vi "Read Temperature Data.vi"(4 "PROM correction Values":u16[](array[numeric]), 6 "I2C Slave Address":u8=119 format="%x", 7 "I2C Channel":u8, 8 "Error In":errorcluster, 11 "LINX Resource in":T1) -> (0 "Error Out":errorcluster, 2 "dT":i32, 3 "LINX Resource out":T1, 5 "Temp":dbl format="%.2g")   [LabVIEW 2014]
uses:
  <vilib>/MakerHub/LINX/Private/Type Defs/LINX Ref.ctl
  <vilib>/MakerHub/LINX/Private/Type Defs/Platform.ctl
  <vilib>/MakerHub/LINX/Private/Type Defs/Interface.ctl
  <vilib>/MakerHub/LINX/Private/Device/Type Defs/LINX Device Config.ctl
  <vilib>/MakerHub/LINX/Private/Device/Type Defs/TCP Config.ctl
  <vilib>/MakerHub/LINX/Private/Device/Type Defs/Channels.ctl
  <vilib>/MakerHub/LINX/Private/Local IO/LinxI2cWrite.vi
  <vilib>/MakerHub/LINX/Public/Utilities/Check Channel.vi
  <vilib>/MakerHub/LINX/Private/Utilties/Generate Error.vi
  <vilib>/MakerHub/LINX/LMH-LINX.lvlib
  <vilib>/MakerHub/LINX/Private/Device/Device.lvlib
panel:
  out "C6":u16
  out "C5":u16
  out "D2":u32
  out "D2 Raw Data Values":u16[](array[numeric])
  # "Data 23-16"
  # "Data 8-15"
  # "Datas 0-7"
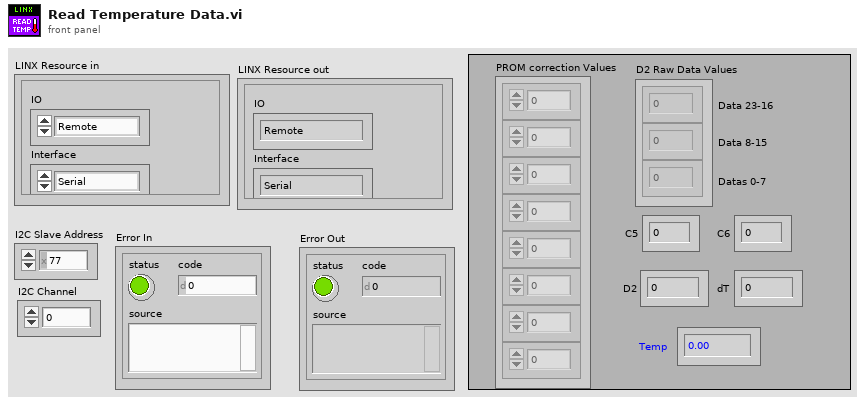
[diagram p1: front panel]
types:
  T1 = typedef "LMH-LINX.lvlib/LINX Ref.ctl" = cluster{"IO":T2, "Interface":T3, "LINX Device Config":T4}
  T2 = typedef "LMH-LINX.lvlib/Platform.ctl" = enum16{"Remote", "Local"}
  T3 = typedef "LMH-LINX.lvlib/Interface.ctl" = enum16{"Serial", "TCP"}
  T4 = typedef "LMH-LINX.lvlib/Device.lvlib/LINX Device Config.ctl" = cluster{"Interface":T3, "COM Port":refnum<visa-resource-name>, "TCP Configuration":T5, "Device Family":u8, "Device ID":u8, "Device Name":string, "TCP Ref":refnum<k5>, "Channels":T6}
  T5 = typedef "LMH-LINX.lvlib/Device.lvlib/TCP Config.ctl" = cluster{"IP Address":string, "Port":u16}
  T6 = typedef "LMH-LINX.lvlib/Channels.ctl" = cluster{"DI":u8[], "DO":u8[], "AI":u8[], "AO":u8[], "PWM":u8[], "QE":u8[], "UART":u8[], "I2C 2":u8[], "SPI":u8[], "CAN":u8[], "Servo":u8[], "AI Ref (V)":dbl, "AI Resolution (Bits)":u8, "AO Ref (V)":dbl, "AO Resolution (Bits)":u8}
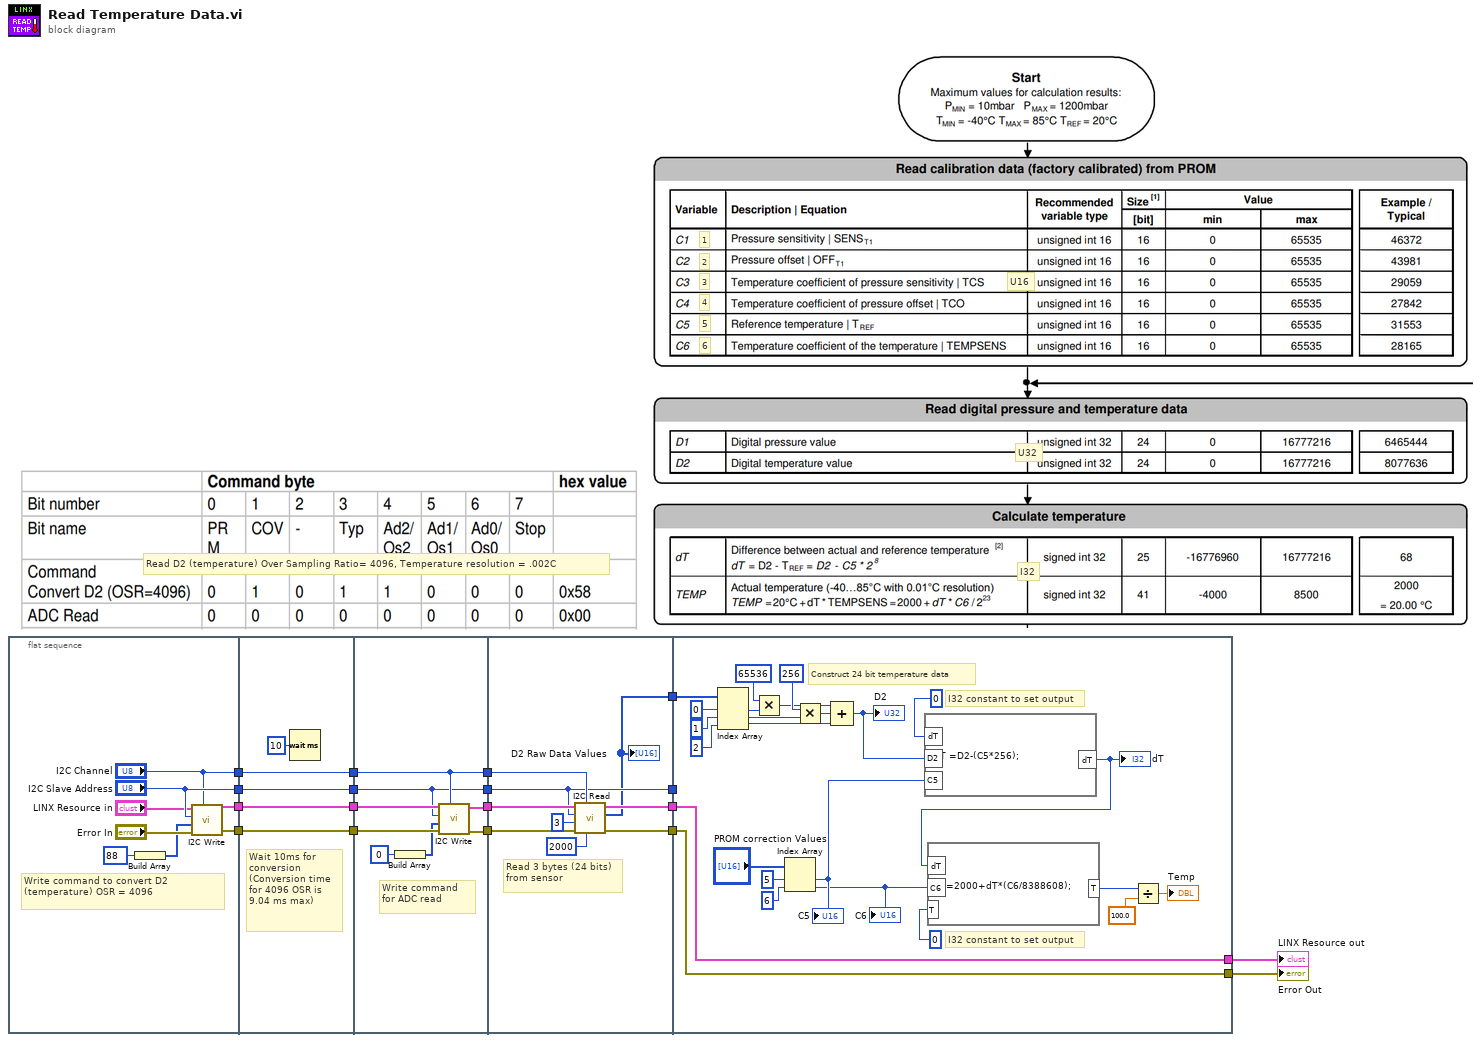
[diagram p0: block diagram]
diagram:
  # "6"
  # "5"
  # "4"
  # "3"
  # "2"
  # "1"
  # "U16"
  # "U32"
  # "I32"
  # "Read D2 (temperature) Over Sampling Ratio= 4096, Temperature resolution = .002C"
  n1 = flat-sequence {
    tunnel: ["I2C Slave Address"] -> w18
    tunnel: ["I2C Channel"] -> w17
    tunnel: [w24] -> w16
    tunnel: [w23] -> w15
    tunnel: w18 -> [w31]
    tunnel: w17 -> [w30]
    tunnel: w16 -> [w29]
    tunnel: w15 -> [w28]
    tunnel: [w31] -> w12
    tunnel: [w30] -> w10
    tunnel: [w29] -> w8
    tunnel: [w28] -> w6
    tunnel: w12 -> [w34]
    tunnel: [w34] -> w11
    tunnel: w10 -> [w35]
    tunnel: [w35] -> w9
    tunnel: w8 -> [w39]
    tunnel: [w37] -> w7
    tunnel: w6 -> [w38]
    tunnel: [w36] -> w5
    tunnel: w11 -> [w41]
    tunnel: w9 -> [w46]
    tunnel: w7 -> [w45]
    tunnel: w5 -> [w44]
    tunnel: [w41] -> w4
    tunnel: [w43] -> w3
    tunnel: [w42] -> w2
    tunnel: [w40] -> w1
    tunnel: [w72] -> w13
    tunnel: [w73] -> w14
    tunnel: w4 -> [_]
    tunnel: w3 -> [w73]
    tunnel: w2 -> [w72]
    tunnel: w1 -> [w71]
    frame #0 {
      # "Write command to convert D2 (temperature) OSR = 4096"
      n2 = Build Array(u8 88) -> (w20:u8[])
      n3 = call <vilib>:"I2C Write.vi"("I2C Channel"="I2C Channel", "Error In"="Error In", "Data"=w20, "I2C Slave Address (0)"="I2C Slave Address", "LINX Resource"="LINX Resource in") -> ("Error Out"=w23:errorcluster, "LINX Resource"=w24:T1)  [unwired: 5 in]
    }
    frame #1 {
      # "Wait 10ms for conversion (Conversion time for 4096 OSR is 9.04 ms max)"
      n4 = Wait (ms)(milliseconds to wait=u32 10) -> ()  [unwired: 1 out]
    }
    frame #2 {
      # "Write command for ADC read"
      n5 = Build Array(u8 0) -> (w32:u8[])
      n6 = call <vilib>:"I2C Write.vi"("I2C Channel"=w35, "Error In"=w38, "Data"=w32, "I2C Slave Address (0)"=w34, "LINX Resource"=w39) -> ("Error Out"=w36:errorcluster, "LINX Resource"=w37:T1)  [unwired: 5 in]
    }
    frame #3 {
      # "Read 3 bytes (24 bits) from sensor"
      n7 = call <vilib>:"I2C Read.vi"("Timeout (1000 ms)"=u16 2000, "I2C Channel"=w46, "Error In"=w44, "Bytes To Read"=u8 3, "I2C Slave Address (0)"=w41, "LINX Resource"=w45) -> ("Error Out"=w43:errorcluster, "Data"=w40:u8[], "LINX Resource"=w42:T1)  [unwired: 3 in]
      "D2 Raw Data Values" <- w40
    }
    frame #4 {
      # "2^23"
      # "2^8"
      # "I32 constant to set output"
      # "I32 constant to set output"
      # "Construct 24 bit temperature data"
      # "2^8"
      n8 = Index Array(array=w71, index #1=0 ("index"), index #2=1 ("index"), index #3=2 ("index")) -> (element #1=w64:u8, element #2=w61:u8, element #3=w58:u8)
      n9 = Multiply(x=u32 65536 ("y"), y=w64) -> (x*y=w59:u32)
      n10 = Index Array(array="PROM correction Values", index #1=5 ("index"), index #2=6 ("index")) -> (element #1=w54:u16, element #2=w51:u16)
      "C5" <- w54
      "C6" <- w51
      n11 = Multiply(x=u32 256 ("y"), y=w61) -> (x*y=w60:u32)
      n12 = Compound Arithmetic op=ADD(w59, w60, w58) -> (w55:u32)
      "D2" <- w55
      n13 = formula code="dT =D2-(C5*256);"("D2"=w55, "C5"=w54, "dT"=0 ("input variable")) -> ("dT"=w52:i32)
      "dT" <- w52
      n14 = formula code="T =2000+dT*(C6/8388608);"("C6"=w51, "T"=0 ("input variable"), "dT"=w52) -> ("T"=w49:i32)
      n15 = Divide(x=w49, y=100.0) -> (x/y=→"Temp":dbl)
    }
  }
  "LINX Resource out" <- w13
  "Error Out" <- w14
